vi "AQT_MEMS_switch_marty_version.vi"() -> ()   [LabVIEW 2012]
uses:
  <userlib>/okFrontPanel/okFrontPanel.lvlib
panel:
  out "initialization return codes":u32[](array[numeric])
  out "set connection return codes\none row for each voltage":u32[][](array[numeric])
  in  "check info when idle":bool
  out "Output data":i32[](array[numeric])
  out "Output addresses":u32[](array[numeric])
  in  "Output Panel":i32(ring)=2 items=["C"=2, "D"=3]
  in  "Input Panel":i32(ring)=11 items=["L"=11]
  in  "Input Number":i32=4 min=2 max=8 step=1
  in  "Output Number":i32=7 min=3 max=7 step=1
  out "Model Number":string
  out "Board ID":string
  in  "Connect":bool
  in  "stop":bool
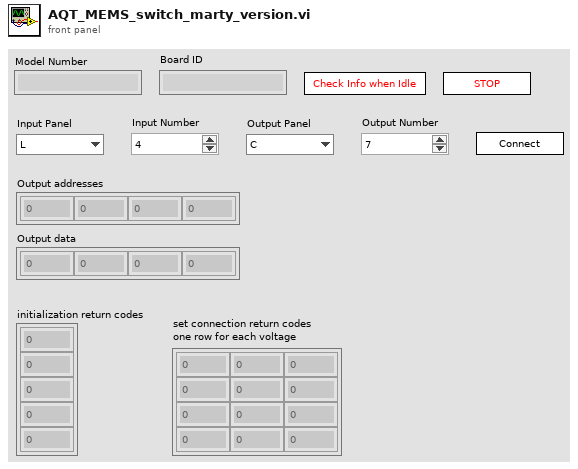
[diagram p1: front panel]
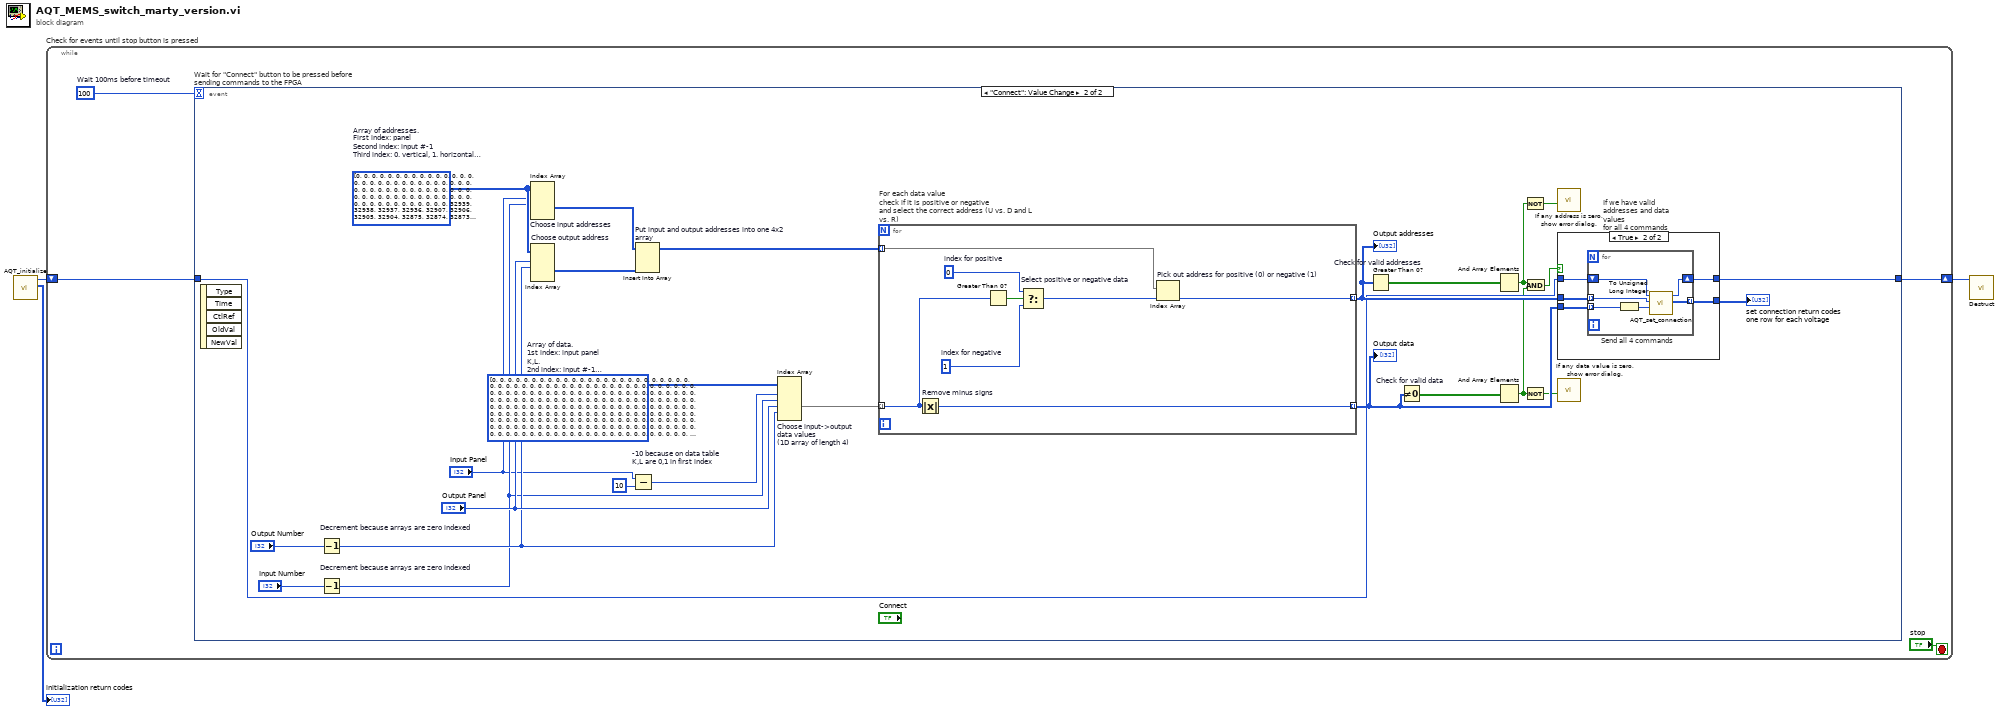
[diagram p0: block diagram]
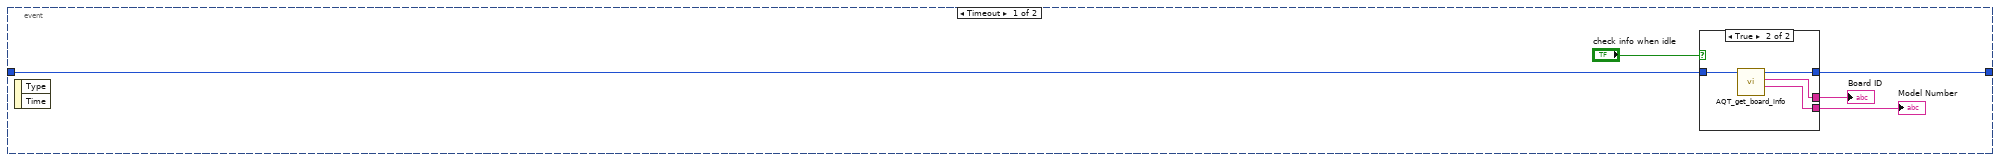
[diagram p2: hidden frame]
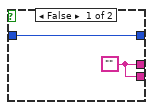
[diagram p3: hidden frame]
diagram:
  n1 = call "AQT_initialize.vi"() -> ("function returns"=→"initialization return codes":u32[], "hnd out"=w3:u32)  [unwired: 10 in]
  n2 = while "Check for events until stop button is pressed" {
    shift-right: [w5] -> w2
    shift-left: w3 -> [w6]
    stop <- "stop" stop-if-true
    w4 = 100  # Wait 100ms before timeout
    n3 = event "Wait for \"Connect\" button to be pressed before sending commands to the FPGA" shown="[1] \"Connect\": Value Change" {
      selector: _ -> [_ _]
      dyn-events: _ -> [_ _]
      timeout: w4 -> [_ _]
      tunnel: w6 -> [w12 w25]
      tunnel: [w11 w24] -> w5
      event Timeout {
        n4 = event-data() -> ()  [unwired: 1 in, 2 out]
        n5 = case shown="True" "check info when idle" {
          tunnel: w12 -> [w14 w18]
          tunnel: [w14 w17] -> w11
          tunnel: [w13 w16] -> w9
          tunnel: [w13 w15] -> w8
          frame False {
            w13 = ""
          }
          frame True {
            n6 = call "AQT_get_board_info.vi"("hnd"=w18) -> ("Model Number"=w15:string, "Board ID"=w16:string, "hnd out"=w17:u32)  [unwired: 8 in]
          }
        }
        "Model Number" <- w8
        "Board ID" <- w9
      }
      event "Connect": Value Change {
        w40 = u32[][][][] [[[[0, 0], [0, 0]], [[0, 0], [0, 0]], [[0, 0], [0, 0]], [[0, 0], [0, 0]], [[0, 0], [0, 0]], [[0, 0], [0, 0]], [[0, 0], [0, 0]], [[0, 0], [0, 0]]], [[[0, 0], [0, 0]], [[0, 0], [0, 0]], [[0, 0], [0, 0]], [[0, 0], [0, 0]], [[0, 0], [0, 0]], [[0, 0], [0, 0]], [[0, 0], [0, 0]], [[0, 0], [0, 0]]], [[[0, 0], [0, 0]], [[0, 0], [0, 0]], [[32939, 32938], [32937, 32936]], [[32907, 32906], [32905, 32904]], [[32875, 32874], [32873, 32872]], [[32843, 32842], [32841, 32840]], [[32811, 32810], [32809, 32808]], [[0, 0], [0, 0]]], [[[0, 0], [0, 0]], [[0, 0], [0, 0]], [[32943, 32942], [0, 32940]], [[32911, 32910], [0, 32908]], [[32879, 32878], [0, 32876]], [[32847, 32846], [0, 32844]], [[32815, 32814], [0, 32812]], [[0, 0], [0, 0]]], [[[0, 0], [0, 0]], [[0, 0], [0, 0]], [[0, 0], [0, 0]], [[0, 0], [0, 0]], [[0, 0], [0, 0]], [[0, 0], [0, 0]], [[0, 0], [0, 0]], [[0, 0], [0, 0]]], [[[0, 0], [0, 0]], [[0, 0], [0, 0]], [[0, 0], [0, 0]], [[0, 0], [0, 0]], [[0, 0], [0, 0]], [[0, 0], [0, 0]], [[0, 0], [0, 0]], [[0, 0], [0, 0]]], [[[0, 0], [0, 0]], [[0, 0], [0, 0]], [[0, 0], [0, 0]], [[0, 0], [0, 0]], [[0, 0], [0, 0]], [[0, 0], [0, 0]], [[0, 0], [0, 0]], [[0, 0], [0, 0]]], [[[0, 0], [0, 0]], [[0, 0], [0, 0]], [[0, 0], [0, 0]], [[0, 0], [0, 0]], [[0, 0], [0, 0]], [[0, 0], [0, 0]], [[0, 0], [0, 0]], [[0, 0], [0, 0]]], [[[0, 0], [0, 0]], [[0, 0], [0, 0]], [[0, 0], [0, 0]], [[0, 0], [0, 0]], [[0, 0], [0, 0]], [[0, 0], [0, 0]], [[0, 0], [0, 0]], [[0, 0], [0, 0]]], [[[0, 0], [0, 0]], [[0, 0], [0, 0]], [[0, 0], [0, 0]], [[0, 0], [0, 0]], [[0, 0], [0, 0]], [[0, 0], [0, 0]], [[0, 0], [0, 0]], [[0, 0], [0, 0]]], [[[0, 0], [0, 0]], [[0, 0], [0, 0]], [[0, 0], [0, 0]], [[0, 0], [0, 0]], [[0, 0], [0, 0]], [[0, 0], [0, 0]], [[0, 0], [0, 0]], [[0, 0], [0, 0]]], [[[0, 0], [0, 0]], [[0, 0], [0, 0]], [[33042, 33043], [33041, 0]], [[33044, 33045], [33046, 33047]], [[0, 0], [0, 0]], [[33076, 33060], [33079, 33062]], [[0, 0], [0, 0]], [[33070, 33082], [33080, 33081]]], [[[0, 0], [0, 0]], [[0, 0], [0, 0]], [[0, 0], [0, 0]], [[0, 0], [0, 0]], [[0, 0], [0, 0]], [[0, 0], [0, 0]], [[0, 0], [0, 0]], [[0, 0], [0, 0]]], [[[0, 0], [0, 0]], [[0, 0], [0, 0]], [[0, 0], [0, 0]], [[0, 0], [0, 0]], [[0, 0], [0, 0]], [[0, 0], [0, 0]], [[0, 0], [0, 0]], [[0, 0], [0, 0]]], [[[0, 0], [0, 0]], [[0, 0], [0, 0]], [[0, 0], [0, 0]], [[0, 0], [0, 0]], [[0, 0], [0, 0]], [[0, 0], [0, 0]], [[0, 0], [0, 0]], [[0, 0], [0, 0]]]]  # Array of addresses. First index: panel Second index: input #-1 Third index: 0. vertical, 1. horizontal Fourth index: 0. positive, 1. negative
        w42 = i32[][][][][] [[[[[0, 0, 0, 0], [0, 0, 0, 0], [0, 0, 0, 0], [0, 0, 0, 0], [0, 0, 0, 0], [0, 0, 0, 0], [0, 0, 0, 0]], [[0, 0, 0, 0], [0, 0, 0, 0], [0, 0, 0, 0], [0, 0, 0, 0], [0, 0, 0, 0], [0, 0, 0, 0], [0, 0, 0, 0]], [[0, 0, 0, 0], [0, 0, 0, 0], [0, 0, 0, 0], [0, 0, 0, 0], [0, 0, 0, 0], [0, 0, 0, 0], [0, 0, 0, 0]], [[0, 0, 0, 0], [0, 0, 0, 0], [0, 0, 0, 0], [0, 0, 0, 0], [0, 0, 0, 0], [0, 0, 0, 0], [0, 0, 0, 0]]], [[[0, 0, 0, 0], [0, 0, 0, 0], [0, 0, 0, 0], [0, 0, 0, 0], [0, 0, 0, 0], [0, 0, 0, 0], [0, 0, 0, 0]], [[0, 0, 0, 0], [0, 0, 0, 0], [0, 0, 0, 0], [0, 0, 0, 0], [0, 0, 0, 0], [0, 0, 0, 0], [0, 0, 0, 0]], [[0, 0, 0, 0], [0, 0, 0, 0], [0, 0, 0, 0], [0, 0, 0, 0], [0, 0, 0, 0], [0, 0, 0, 0], [0, 0, 0, 0]], [[0, 0, 0, 0], [0, 0, 0, 0], [0, 0, 0, 0], [0, 0, 0, 0], [0, 0, 0, 0], [0, 0, 0, 0], [0, 0, 0, 0]]], [[[0, 0, 0, 0], [0, 0, 0, 0], [0, 0, 0, 0], [0, 0, 0, 0], [0, 0, 0, 0], [0, 0, 0, 0], [0, 0, 0, 0]], [[0, 0, 0, 0], [0, 0, 0, 0], [0, 0, 0, 0], [0, 0, 0, 0], [0, 0, 0, 0], [0, 0, 0, 0], [0, 0, 0, 0]], [[0, 0, 0, 0], [0, 0, 0, 0], [0, 0, 0, 0], [0, 0, 0, 0], [0, 0, 0, 0], [0, 0, 0, 0], [0, 0, 0, 0]], [[0, 0, 0, 0], [0, 0, 0, 0], [0, 0, 0, 0], [0, 0, 0, 0], [0, 0, 0, 0], [0, 0, 0, 0], [0, 0, 0, 0]]], [[[0, 0, 0, 0], [0, 0, 0, 0], [0, 0, 0, 0], [0, 0, 0, 0], [0, 0, 0, 0], [0, 0, 0, 0], [0, 0, 0, 0]], [[0, 0, 0, 0], [0, 0, 0, 0], [0, 0, 0, 0], [0, 0, 0, 0], [0, 0, 0, 0], [0, 0, 0, 0], [0, 0, 0, 0]], [[0, 0, 0, 0], [0, 0, 0, 0], [0, 0, 0, 0], [0, 0, 0, 0], [0, 0, 0, 0], [0, 0, 0, 0], [0, 0, 0, 0]], [[0, 0, 0, 0], [0, 0, 0, 0], [0, 0, 0, 0], [0, 0, 0, 0], [0, 0, 0, 0], [0, 0, 0, 0], [0, 0, 0, 0]]], [[[0, 0, 0, 0], [0, 0, 0, 0], [0, 0, 0, 0], [0, 0, 0, 0], [0, 0, 0, 0], [0, 0, 0, 0], [0, 0, 0, 0]], [[0, 0, 0, 0], [0, 0, 0, 0], [0, 0, 0, 0], [0, 0, 0, 0], [0, 0, 0, 0], [0, 0, 0, 0], [0, 0, 0, 0]], [[0, 0, 0, 0], [0, 0, 0, 0], [0, 0, 0, 0], [0, 0, 0, 0], [0, 0, 0, 0], [0, 0, 0, 0], [0, 0, 0, 0]], [[0, 0, 0, 0], [0, 0, 0, 0], [0, 0, 0, 0], [0, 0, 0, 0], [0, 0, 0, 0], [0, 0, 0, 0], [0, 0, 0, 0]]], [[[0, 0, 0, 0], [0, 0, 0, 0], [0, 0, 0, 0], [0, 0, 0, 0], [0, 0, 0, 0], [0, 0, 0, 0], [0, 0, 0, 0]], [[0, 0, 0, 0], [0, 0, 0, 0], [0, 0, 0, 0], [0, 0, 0, 0], [0, 0, 0, 0], [0, 0, 0, 0], [0, 0, 0, 0]], [[0, 0, 0, 0], [0, 0, 0, 0], [0, 0, 0, 0], [0, 0, 0, 0], [0, 0, 0, 0], [0, 0, 0, 0], [0, 0, 0, 0]], [[0, 0, 0, 0], [0, 0, 0, 0], [0, 0, 0, 0], [0, 0, 0, 0], [0, 0, 0, 0], [0, 0, 0, 0], [0, 0, 0, 0]]], [[[0, 0, 0, 0], [0, 0, 0, 0], [0, 0, 0, 0], [0, 0, 0, 0], [0, 0, 0, 0], [0, 0, 0, 0], [0, 0, 0, 0]], [[0, 0, 0, 0], [0, 0, 0, 0], [0, 0, 0, 0], [0, 0, 0, 0], [0, 0, 0, 0], [0, 0, 0, 0], [0, 0, 0, 0]], [[0, 0, 0, 0], [0, 0, 0, 0], [0, 0, 0, 0], [0, 0, 0, 0], [0, 0, 0, 0], [0, 0, 0, 0], [0, 0, 0, 0]], [[0, 0, 0, 0], [0, 0, 0, 0], [0, 0, 0, 0], [0, 0, 0, 0], [0, 0, 0, 0], [0, 0, 0, 0], [0, 0, 0, 0]]], [[[0, 0, 0, 0], [0, 0, 0, 0], [0, 0, 0, 0], [0, 0, 0, 0], [0, 0, 0, 0], [0, 0, 0, 0], [0, 0, 0, 0]], [[0, 0, 0, 0], [0, 0, 0, 0], [0, 0, 0, 0], [0, 0, 0, 0], [0, 0, 0, 0], [0, 0, 0, 0], [0, 0, 0, 0]], [[0, 0, 0, 0], [0, 0, 0, 0], [0, 0, 0, 0], [0, 0, 0, 0], [0, 0, 0, 0], [0, 0, 0, 0], [0, 0, 0, 0]], [[0, 0, 0, 0], [0, 0, 0, 0], [0, 0, 0, 0], [0, 0, 0, 0], [0, 0, 0, 0], [0, 0, 0, 0], [0, 0, 0, 0]]]], [[[[0, 0, 0, 0], [0, 0, 0, 0], [0, 0, 0, 0], [0, 0, 0, 0], [0, 0, 0, 0], [0, 0, 0, 0], [0, 0, 0, 0]], [[0, 0, 0, 0], [0, 0, 0, 0], [0, 0, 0, 0], [0, 0, 0, 0], [0, 0, 0, 0], [0, 0, 0, 0], [0, 0, 0, 0]], [[0, 0, 0, 0], [0, 0, 0, 0], [0, 0, 0, 0], [0, 0, 0, 0], [0, 0, 0, 0], [0, 0, 0, 0], [0, 0, 0, 0]], [[0, 0, 0, 0], [0, 0, 0, 0], [0, 0, 0, 0], [0, 0, 0, 0], [0, 0, 0, 0], [0, 0, 0, 0], [0, 0, 0, 0]]], [[[0, 0, 0, 0], [0, 0, 0, 0], [0, 0, 0, 0], [0, 0, 0, 0], [0, 0, 0, 0], [0, 0, 0, 0], [0, 0, 0, 0]], [[0, 0, 0, 0], [0, 0, 0, 0], [0, 0, 0, 0], [0, 0, 0, 0], [0, 0, 0, 0], [0, 0, 0, 0], [0, 0, 0, 0]], [[0, 0, 0, 0], [0, 0, 0, 0], [-652, 530, 6340, -3200], [-460, 320, 6300, -3200], [200, 342, 6260, -3400], [510, 310, 6200, -3200], [0, 0, 0, 0]], [[0, 0, 0, 0], [0, 0, 0, 0], [-640, -422, 6960, -4060], [-458, -270, 6380, -2960], [200, -290, 6200, -3100], [512, -244, 6180, -3120], [0, 0, 0, 0]]], [[[0, 0, 0, 0], [0, 0, 0, 0], [0, 0, 0, 0], [0, 0, 0, 0], [0, 0, 0, 0], [0, 0, 0, 0], [0, 0, 0, 0]], [[0, 0, 0, 0], [0, 0, 0, 0], [0, 0, 0, 0], [0, 0, 0, 0], [0, 0, 0, 0], [0, 0, 0, 0], [0, 0, 0, 0]], [[0, 0, 0, 0], [0, 0, 0, 0], [656, 604, 3860, 3620], [-466, 318, 3600, 3680], [176, 352, 3880, 3520], [494, 400, 3760, 3740], [670, 720, 3700, 3400]], [[0, 0, 0, 0], [0, 0, 0, 0], [0, 0, 0, 0], [0, 0, 0, 0], [0, 0, 0, 0], [0, 0, 0, 0], [0, 0, 0, 0]]], [[[0, 0, 0, 0], [0, 0, 0, 0], [0, 0, 0, 0], [0, 0, 0, 0], [0, 0, 0, 0], [0, 0, 0, 0], [0, 0, 0, 0]], [[0, 0, 0, 0], [0, 0, 0, 0], [0, 0, 0, 0], [0, 0, 0, 0], [0, 0, 0, 0], [0, 0, 0, 0], [0, 0, 0, 0]], [[0, 0, 0, 0], [0, 0, 0, 0], [-680, 680, 3760, -3340], [-492, 284, 3460, -3440], [362, 228, 3660, -3460], [428, 534, 3640, -3260], [716, 710, 3580, -3600]], [[0, 0, 0, 0], [0, 0, 0, 0], [-668, -426, 3640, -3280], [-478, -276, 3720, -3280], [246, -286, 3700, -3120], [534, -236, 3600, -3200], [716, -446, 3880, -3360]]], [[[0, 0, 0, 0], [0, 0, 0, 0], [0, 0, 0, 0], [0, 0, 0, 0], [0, 0, 0, 0], [0, 0, 0, 0], [0, 0, 0, 0]], [[0, 0, 0, 0], [0, 0, 0, 0], [0, 0, 0, 0], [0, 0, 0, 0], [0, 0, 0, 0], [0, 0, 0, 0], [0, 0, 0, 0]], [[0, 0, 0, 0], [0, 0, 0, 0], [0, 0, 0, 0], [0, 0, 0, 0], [0, 0, 0, 0], [0, 0, 0, 0], [0, 0, 0, 0]], [[0, 0, 0, 0], [0, 0, 0, 0], [0, 0, 0, 0], [0, 0, 0, 0], [0, 0, 0, 0], [0, 0, 0, 0], [0, 0, 0, 0]]], [[[0, 0, 0, 0], [0, 0, 0, 0], [0, 0, 0, 0], [0, 0, 0, 0], [0, 0, 0, 0], [0, 0, 0, 0], [0, 0, 0, 0]], [[0, 0, 0, 0], [0, 0, 0, 0], [0, 0, 0, 0], [0, 0, 0, 0], [0, 0, 0, 0], [0, 0, 0, 0], [0, 0, 0, 0]], [[0, 0, 0, 0], [0, 0, 0, 0], [-614, 556, -4500, -3000], [-442, 432, -4480, -3400], [-316, 488, -4560, -3380], [562, 416, -4560, -3040], [730, 730, -3200, -4600]], [[0, 0, 0, 0], [0, 0, 0, 0], [-624, -542, -4520, -3120], [-430, -316, -4560, -2940], [328, -350, -4600, -3000], [550, -376, -4800, -3140], [738, -740, -4380, -3240]]], [[[0, 0, 0, 0], [0, 0, 0, 0], [0, 0, 0, 0], [0, 0, 0, 0], [0, 0, 0, 0], [0, 0, 0, 0], [0, 0, 0, 0]], [[0, 0, 0, 0], [0, 0, 0, 0], [0, 0, 0, 0], [0, 0, 0, 0], [0, 0, 0, 0], [0, 0, 0, 0], [0, 0, 0, 0]], [[0, 0, 0, 0], [0, 0, 0, 0], [0, 0, 0, 0], [0, 0, 0, 0], [0, 0, 0, 0], [0, 0, 0, 0], [0, 0, 0, 0]], [[0, 0, 0, 0], [0, 0, 0, 0], [0, 0, 0, 0], [0, 0, 0, 0], [0, 0, 0, 0], [0, 0, 0, 0], [0, 0, 0, 0]]], [[[0, 0, 0, 0], [0, 0, 0, 0], [0, 0, 0, 0], [0, 0, 0, 0], [0, 0, 0, 0], [0, 0, 0, 0], [0, 0, 0, 0]], [[0, 0, 0, 0], [0, 0, 0, 0], [0, 0, 0, 0], [0, 0, 0, 0], [0, 0, 0, 0], [0, 0, 0, 0], [0, 0, 0, 0]], [[0, 0, 0, 0], [0, 0, 0, 0], [-570, 300, -6380, -3320], [-422, 246, -4760, -3880], [280, 262, -6800, -3860], [530, 230, -6880, -3720], [0, 0, 0, 0]], [[0, 0, 0, 0], [0, 0, 0, 0], [-620, -600, -6960, -4060], [-410, -360, -6900, -3840], [290, -340, -6740, -3420], [560, -310, -7200, -4240], [0, 0, 0, 0]]]]]  # Array of data. 1st index: input panel K,L. 2nd index: input #-1 3rd index: output panel A,B,C,D,E,F,G,H 4th index: output #-1 5th index: input U/D, input L/R, output U/D, output L/R Positive values indicate U and L, negative values indicate D and R.
        n7 = event-data() -> ()  [unwired: 1 in, 5 out]
        n8 = Decrement "Decrement because arrays are zero indexed"(x="Output Number") -> (x-1=w38:i32)
        n9 = Decrement "Decrement because arrays are zero indexed"(x="Input Number") -> (x-1=w36:i32)
        n10 = Index Array "Choose input addresses"(array=w40, index (dim 0)="Input Panel", index (dim 1)=w36) -> (element=w33:u32[][])  [unwired: 2 in]
        n11 = Index Array "Choose output address"(array=w40, index (dim 0)="Output Panel", index (dim 1)=w38) -> (element=w32:u32[][])  [unwired: 2 in]
        n12 = Subtract "-10 because on data table\nK,L are 0,1 in first index"(x="Input Panel", y=10) -> (x-y=w34:i32)
        n13 = Insert Into Array "Put input and output addresses into one 4x2 array"(array=w33, new element=w32) -> (w31:u32[][])  [unwired: 2 in]
        n14 = Index Array "Choose input->output\ndata values\n(1D array of length 4)"(array=w42, index (dim 0)=w34, index (dim 1)=w36, index (dim 2)="Output Panel", index (dim 3)=w38) -> (element=w41:i32[])  [unwired: 1 in]
        n15 = for "For each data value\ncheck if it is positive or negative\nand select the correct address (U vs. D and L vs. R)" {
          tunnel: w41 -> [w58] mode=indexing
          tunnel: w31 -> [w63] mode=indexing
          tunnel: [w59] -> w27 mode=indexing
          tunnel: [w57] -> w26 mode=indexing
          w61 = 1  # index for negative
          w62 = 0  # index for positive
          n16 = Absolute Value "Remove minus signs"(x=w58) -> (abs(x)=w57:i32)
          n17 = Greater Than 0?(x=w58) -> (x > 0?=w64:bool)
          n18 = Select "Select positive or negative data"(t=w62, s=w64, f=w61) -> (s? t:f=w60:i32)
          n19 = Index Array "Pick out address for positive (0) or negative (1)"(array=w63, index=w60) -> (element=w59:u32)
        }
        "Output addresses" <- w27
        "Output data" <- w26
        n20 = Greater Than 0? "Check for valid addresses"(x=w27) -> (x > 0?=w30:bool[])
        n21 = Not Equal To 0? "Check for valid data"(x=w26) -> (x != 0?=w29:bool[])
        n22 = And Array Elements(Boolean array=w30) -> (logical AND=w22:bool)
        n23 = And Array Elements(Boolean array=w29) -> (logical AND=w20:bool)
        n24 = Not(x=w22) -> (.not. x?=w21:bool)
        n25 = Not(x=w20) -> (.not. x?=w19:bool)
        n26 = And(x=w22, y=w20) -> (x .and. y?=w28:bool)
        n27 = call "If any address is zero, show error dialog."("Enable"=w21) -> ()  [unwired: 9 in, 2 out]
        n28 = case "If we have valid addresses and data values\nfor all 4 commands" shown="True" w28 {
          tunnel: w27 -> [_ w50]
          tunnel: w26 -> [_ w49]
          tunnel: w25 -> [w45 w48]
          tunnel: [w45 w47] -> w24
          tunnel: [_ w46] -> w23
          frame False {
          }
          frame True {
            n29 = for "Send all 4 commands" {
              tunnel: w50 -> [w54] mode=indexing
              tunnel: w49 -> [w53] mode=indexing
              shift-right: [w55] -> w47
              shift-left: w48 -> [w56]
              tunnel: [w51] -> w46 mode=indexing
              n30 = To Unsigned Long Integer(number=w53) -> (unsigned 32bit integer=w52:u32)
              n31 = call "AQT_set_connection.vi"("data"=w52, "address"=w54, "hnd"=w56) -> ("return codes"=w51:u32[], "hnd out"=w55:u32)  [unwired: 7 in]
            }
          }
        }
        "set connection return codes\none row for each voltage" <- w23
        n32 = call "If any data value is zero, show error dialog."("Enable"=w19) -> ()  [unwired: 9 in, 2 out]
      }
    }
  }
  n33 = call <userlib>:"Destruct.vi"("hnd"=w2) -> ()  [unwired: 10 in, 1 out]
